vi "PLL_PID_WithoutPIDToolkit.vi"() -> ()   [LabVIEW 2019]
uses:
  <vilib>/measure/matone.llb/Extract Single Tone Information 1 Chan.vi
  <vilib>/measure/NI_MABase.lvlib
  <vilib>/measure/NI_MAPro.lvlib
  <vilib>/Analysis/NI_AALPro.lvlib
panel:
  in  "stop":bool
  out "Waveform Graph":waveform(dbl)[](graph)=[{"t0"=timestamp(0 s since 1904-01-01), "dt"=0.001, "Y"=array[1000 elements]}, {"t0"=timestamp(0 s since 1904-01-01), "dt"=0.001, "Y"=array[1000 elements]}]
  in  "PID_Frequency":T1={"proportional gain (Kc)"=0.9, "integral time (Ti, min)"=0.0008, "derivative time (Td, min)"=0.0} {"derivative time (Td, min)" format="%.3f"; "integral time (Ti, min)" format="%.5f"; "proportional gain (Kc)" format="%.3f"}
  out "Current Frequency [Hz]":dbl=6.999999983966189 format="%.2f"
  in  "Desired Frequency [Hz]":dbl=7.0 format="%_6f"
  in  "PID_Phase":T1={"proportional gain (Kc)"=0.1, "integral time (Ti, min)"=0.0008, "derivative time (Td, min)"=0.0} {"derivative time (Td, min)" format="%.3f"; "integral time (Ti, min)" format="%.5f"; "proportional gain (Kc)" format="%.3f"}
  in  "sampling info":cluster{"Fs":dbl, "#s":dbl}={"Fs"=1000.0, "#s"=1000.0} {"Fs" format="%.2p"}
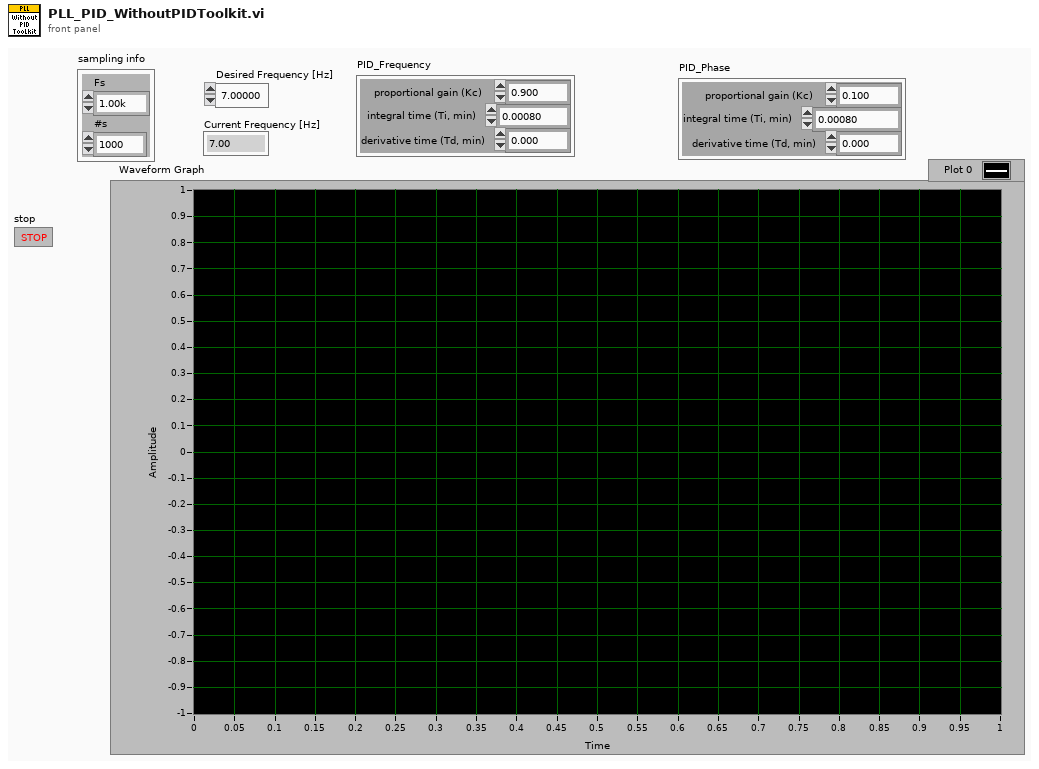
[diagram p1: front panel]
types:
  T1 = cluster{"proportional gain (Kc)":dbl, "integral time (Ti, min)":dbl, "derivative time (Td, min)":dbl}
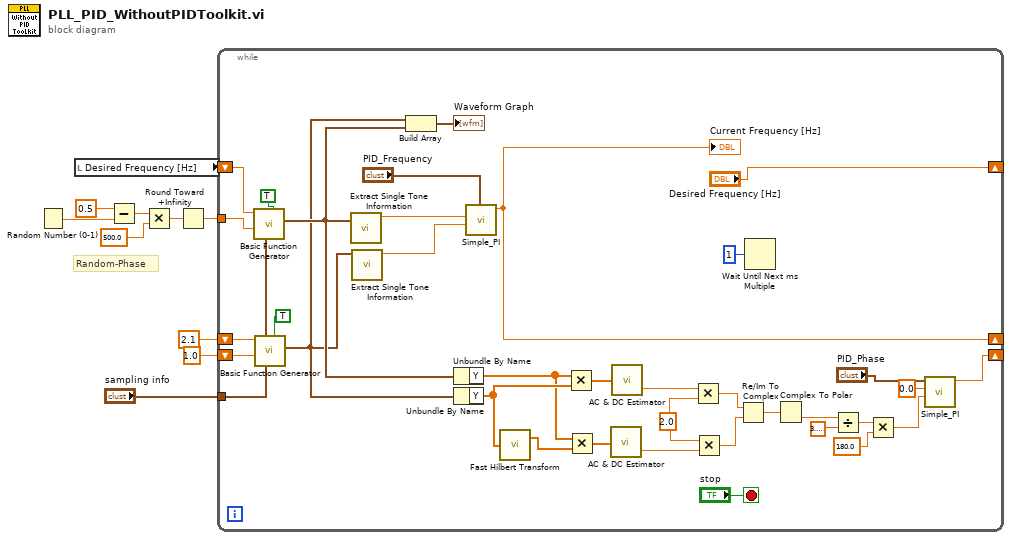
[diagram p0: block diagram]
diagram:
  # "Random-Phase"
  n1 = Random Number (0-1)() -> (number: 0 to 1=w8:dbl)
  n2 = local read "Desired Frequency [Hz]"() -> (w1:dbl)
  n3 = Subtract(x=0.5, y=w8) -> (x-y=w2:dbl)
  n4 = Multiply(x=w2, y=500.0) -> (x*y=w5:dbl)
  n5 = Round Toward +Infinity(x=w5) -> (ceil(x): smallest int >= x=w4:dbl)
  n6 = while {
    tunnel: "sampling info" -> [w46]
    shift-right: [w11] -> _
    shift-left: 1.0 -> [w27]
    tunnel: w4 -> [w19]
    shift-right: [w15] -> _
    shift-left: 2.1 ("f") -> [w41]
    shift-right: ["Desired Frequency [Hz]"] -> _
    shift-left: w1 -> [w21]
    stop <- "stop" stop-if-true
    w25 = 2.0 ("x")
    n7 = call <vilib>:"Basic Function Generator.vi"("reset signal"=TRUE, "sampling info"=w46, "phase"=w19, "frequency"=w21) -> ("signal out"=w24:waveform(dbl))  [unwired: 5 in, 2 out]
    n8 = call <vilib>:"Basic Function Generator.vi"("reset signal"=TRUE, "sampling info"=w46, "phase"=w27, "frequency"=w41) -> ("signal out"=w23:waveform(dbl))  [unwired: 5 in, 2 out]
    n9 = call-poly <vilib>:"Extract Single Tone Information.vi"("time signal in"=w24) -> ("detected frequency"=w17:dbl)  [unwired: 5 in, 5 out]
    n10 = call-poly <vilib>:"Extract Single Tone Information.vi"("time signal in"=w23) -> ("detected frequency"=w16:dbl)  [unwired: 5 in, 5 out]
    n11 = Build Array(w23, w24) -> (→"Waveform Graph":waveform(dbl)[])
    n12 = Unbundle By Name(w24) -> ("Y"=w38:dbl[])
    n13 = Unbundle By Name(w23) -> ("Y"=w40:dbl[])
    n14 = call "Simple_PI.vi"("Current"=w16, "Desired"=w17, "input cluster"="PID_Frequency") -> ("Y"=w15:dbl)  [unwired: 8 in]
    "Current Frequency [Hz]" <- w15
    n15 = call <vilib>:"Fast Hilbert Transform.vi"("X"=w40) -> ("Hilbert{X}"=w39:dbl[])  [unwired: 1 out]
    n16 = Multiply(x=w38, y=w40) -> (x*y=w37:dbl[])
    n17 = Multiply(x=w38, y=w39) -> (x*y=w36:dbl[])
    n18 = call <vilib>:"AC & DC Estimator.vi"("Signal (V)"=w36) -> ("DC estimate (V)"=w35:dbl)  [unwired: 1 out]
    n19 = call <vilib>:"AC & DC Estimator.vi"("Signal (V)"=w37) -> ("DC estimate (V)"=w26:dbl)  [unwired: 1 out]
    n20 = Multiply(x=w26, y=w25) -> (x*y=w29:dbl)
    n21 = Multiply(x=w25, y=w35) -> (x*y=w28:dbl)
    n22 = Re/Im To Complex(1:w28, 2:w29) -> (0:w30:cdb)
    n23 = Wait Until Next ms Multiple(millisecond multiple=u32 1) -> ()  [unwired: 1 out]
    n24 = Complex To Polar(r * e^(i*theta)=w30) -> (theta=w31:dbl)  [unwired: 1 out]
    n25 = Divide(x=w31, y=3.141592653589793) -> (x/y=w33:dbl)
    n26 = Multiply(x=w33, y=180.0) -> (x*y=w12:dbl)
    n27 = call "Simple_PI.vi"("Current"=w12, "Desired"=0.0, "input cluster"="PID_Phase") -> ("Y"=w11:dbl)  [unwired: 8 in]
  }
